vi "AutoPlaySelection.vi"(1 "Selected Auto Play":u16, 2 "Auto Plays":string[](array[string])) -> (0 "Autonomous Commands":string)   [LabVIEW 2019]
doc: "This VI reads the selected autonomous play text file from the roboRIO file system."
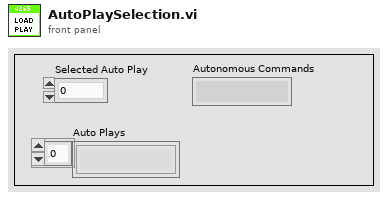
[diagram p1: front panel]
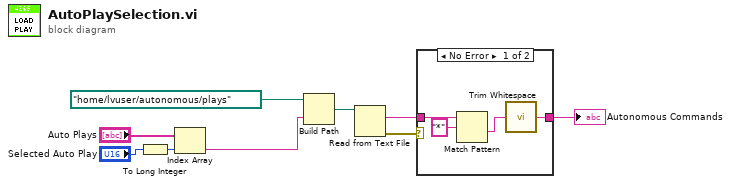
[diagram p0: block diagram]
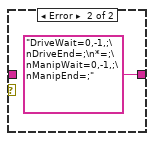
[diagram p2: hidden frame]
diagram:
  n1 = To Long Integer(number="Selected Auto Play") -> (32bit integer=w5:i32)
  n2 = Index Array(array="Auto Plays", index=w5) -> (element=w6:string)
  n3 = Build Path(base path=path "/home/lvuser/autonomous/plays" ("path"), name or relative path=w6) -> (appended path=w4:path)
  n4 = Read from Text File(file (use dialog)=w4) -> (text=w2:string, error out=w3:errorcluster)  [unwired: 3 in, 2 out]
  n5 = case shown="No Error" w3 {
    tunnel: w2 -> [w13 _]
    tunnel: [w12 "DriveWait=0,-1,;\nDriveEnd=;\n*=;\nManipWait=0,-1,;\nManipEnd=;"] -> w1
    frame No Error {
      n6 = Match Pattern(string=w13, regular expression="*") -> (after substring=w11:string)  [unwired: 1 in, 3 out]
      n7 = call <vilib>:"Trim Whitespace.vi"("string"=w11) -> ("trimmed string"=w12:string)  [unwired: 1 in]
    }
    frame Error {
    }
  }
  "Autonomous Commands" <- w1
